vi "Quick Read (No Objects).vi"(8 "error in (no error)":errorcluster, 11 "Fluke Multimeter In":T1 {"function (0:volts DC)" items=["volts DC", "volts AC", "2-wire k.ohms", "4-wire k.ohms", "mA DC", "mA AC"]; "range (0:auto)" items=["autorange", "200mV, 200 ohms", "2V, 2 kohms", "20V, 20 kohms", "200V, 200 kohms", "1000Vdc, 700 Vac, 2 Mohms", "20 Mohms"]; "rate (0:slow)" items=["slow", "medium", "fast"]; "trigger mode (0:internal)" items=["internal - continuous trigger", "external - rear panel trigger with delay", "external - bus trigger with delay", "external - rear panel trigger", "external - bus trigger"]}) -> (0 "error out":errorcluster, 1 "unit":string, 2 "measurement":dbl format="%^.6e", 3 "Fluke Multimeter Out":T1 {"function (0:volts DC)" items=["volts DC", "volts AC", "2-wire k.ohms", "4-wire k.ohms", "mA DC", "mA AC"]; "range (0:auto)" items=["autorange", "200mV, 200 ohms", "2V, 2 kohms", "20V, 20 kohms", "200V, 200 kohms", "1000Vdc, 700 Vac, 2 Mohms", "20 Mohms"]; "rate (0:slow)" items=["slow", "medium", "fast"]; "trigger mode (0:internal)" items=["internal - continuous trigger", "external - rear panel trigger with delay", "external - bus trigger with delay", "external - rear panel trigger", "external - bus trigger"]})   [LabVIEW 2017]
doc: "Performs a quick read. Must use Init & Config Method before use."
uses:
  Global/GPIB Numbers.vi
  Fluke 8840/Fluke 8840.lvlib
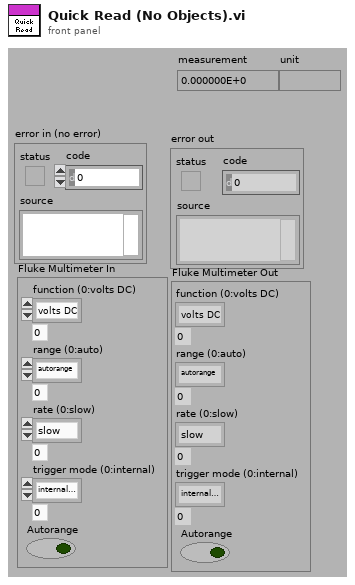
[diagram p1: front panel]
types:
  T1 = cluster{"function (0:volts DC)":u16, "range (0:auto)":u16, "rate (0:slow)":u16, "trigger mode (0:internal)":u16, "Autorange":bool}
  T2 = typedef "GPIB Type Def.ctl" = cluster{"Name":string, "bus":dbl, "GPIB":dbl, "GPIB as string":string, "byte":i32, "VISA Resource Name":refnum<visa-resource-name>}
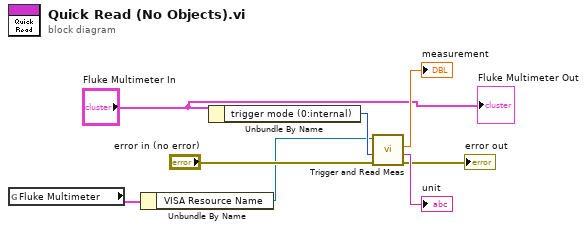
[diagram p0: block diagram]
diagram:
  n1 = global read "GPIB Numbers.vi" "Fluke Multimeter"() -> (w5:T2)
  n2 = Unbundle By Name(w5) -> ("VISA Resource Name"=w2:refnum<visa-resource-name>)
  n3 = Unbundle By Name("Fluke Multimeter In") -> ("trigger mode (0:internal)"=w8:u16)
  n4 = call "Trigger and Read Meas.vi"("error in (no error)"="error in (no error)", "trigger mode (0:internal)"=w8, "VISA resource name"=w2) -> ("error out"=→"error out":errorcluster, "unit"=→"unit":string, "measurement"=→"measurement":dbl)  [unwired: 5 in, 1 out]
  "Fluke Multimeter Out" <- "Fluke Multimeter In"
